vi "Insert Device Panel.vi"(8 "error in (no error)":errorcluster, 9 "Close Event":refnum<user-event>, 10 "Device Panel":refnum<vi>, 11 "Device":refnum<class "Device.lvclass">) -> (0 "error out":errorcluster)   [LabVIEW 2020, in "HAL Config.lvlib" / "HAL Editor.lvclass"]
uses:
  HAL Editor.lvclass
  build/ppl/lv-hal.lvlibp/Device/Device.lvclass
  build/ppl/lv-hal.lvlibp/Device/Editor Event Data.ctl
  Editor UI Terminals.ctl
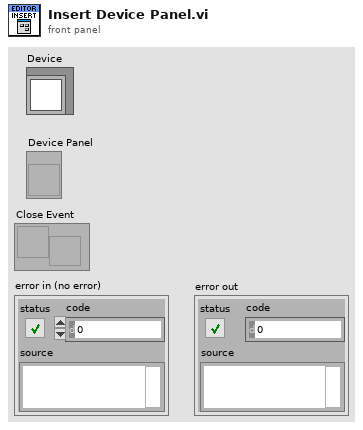
[diagram p1: front panel]
types:
  T1 = typedef "HAL Config.lvlib/HAL Editor.lvclass/Editor UI Terminals.ctl" = i32
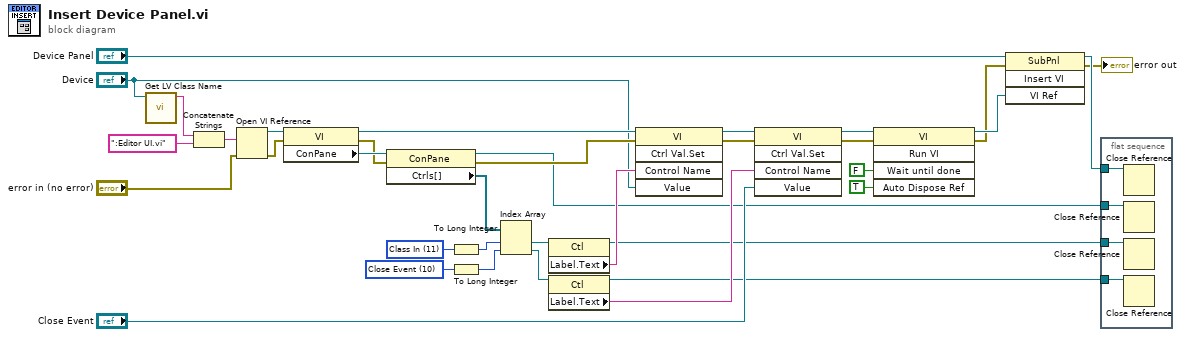
[diagram p0: block diagram]
diagram:
  w27 = T1 10 items=["Close Event"=10, "Class In"=11] ("Editor UI Terminals")
  w28 = T1 11 items=["Close Event"=10, "Class In"=11] ("Editor UI Terminals")
  n1 = call <vilib>:"Get LV Class Name.vi"("object"="Device") -> ("class name"=w35:string)  [unwired: 9 in, 1 out]
  n2 = Concatenate Strings(w35, ":Editor UI.vi" ("string")) -> (w33:string)
  n3 = Open VI Reference(vi path=w33, error in (no error)="error in (no error)") -> (vi reference=w32:refnum<vi>, error out=w31:errorcluster)  [unwired: 4 in]
  n4 = property class="VI"(reference=w32, error in=w31) -> (reference out=w22:refnum<vi>, error out=w17:errorcluster, "ConPane"=w30:refnum<vi>)
  n5 = property class="ConPane"(reference=w30, error in=w17) -> (reference out=w11:refnum<vi>, error out=w16:errorcluster, "Ctrls[]"=w29:refnum<vi>[])
  n6 = To Long Integer(number=w28) -> (32bit integer=w26:T1)
  n7 = To Long Integer(number=w27) -> (32bit integer=w25:T1)
  n8 = Index Array(array=w29, index #1=w26, index #2=w25) -> (element #1=w24:refnum<vi>, element #2=w23:refnum<vi>)
  n9 = property class="Ctl"(reference=w24) -> (reference out=w12:refnum<vi>, "Label.Text"=w21:string)  [unwired: 1 in, 1 out]
  n10 = property class="Ctl"(reference=w23) -> (reference out=w13:refnum<vi>, "Label.Text"=w19:string)  [unwired: 1 in, 1 out]
  n11 = invoke class="VI" method="Ctrl Val.Set"(reference=w22, error in=w16, "Control Name"=w21, "Value"="Device") -> (reference out=w20:refnum<vi>, error out=w15:errorcluster)  [unwired: 1 in, 3 out]
  n12 = invoke class="VI" method="Ctrl Val.Set"(reference=w20, error in=w15, "Control Name"=w19, "Value"="Close Event") -> (reference out=w9:refnum<vi>, error out=w8:errorcluster)  [unwired: 1 in, 3 out]
  n13 = invoke class="VI" method="Run VI"(reference=w9, error in=w8, "Wait until done"=FALSE ("Wait Until Done"), "Auto Dispose Ref"=TRUE ("Auto Dispose Reference")) -> (reference out=w5:refnum<vi>, error out=w4:errorcluster)  [unwired: 1 in, 3 out]
  n14 = invoke class="SubPnl" method="Insert VI"(reference="Device Panel", error in=w4, "VI Ref"=w5) -> (reference out=w3:refnum<vi>, error out=→"error out":errorcluster)  [unwired: 1 in, 2 out]
  n15 = flat-sequence {
    tunnel: w13 -> [w39]
    tunnel: w12 -> [w38]
    tunnel: w11 -> [w37]
    tunnel: w3 -> [w36]
    frame #0 {
      n16 = Close Reference(reference=w36) -> ()  [unwired: 1 in, 1 out]
      n17 = Close Reference(reference=w37) -> ()  [unwired: 1 in, 1 out]
      n18 = Close Reference(reference=w38) -> ()  [unwired: 1 in, 1 out]
      n19 = Close Reference(reference=w39) -> ()  [unwired: 1 in, 1 out]
    }
  }
